vi "OnshapeAngles.vi"   [LabVIEW 2022 SP3]
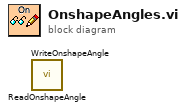
[diagram p0: block diagram]
diagram:
  n1 = call "ReadOnshapeAngle.vi"() -> ()  [unwired: 8 in, 4 out]
  n2 = call "WriteOnshapeAngle.vi"() -> ()  [unwired: 12 in]
